vi "chart axis set display units visible.vi"(8 "error in (no error)":errorcluster, 10 "visible":u8, 11 "axis":u32) -> (0 "error out":errorcluster)   [LabVIEW 8.6]
doc: "void chart_axis_set_display_units_visible(lxw_chart_axis axis, uint8_t visible);"
uses:
  pending_lvxlsxwriter/xlsxwriter.dll
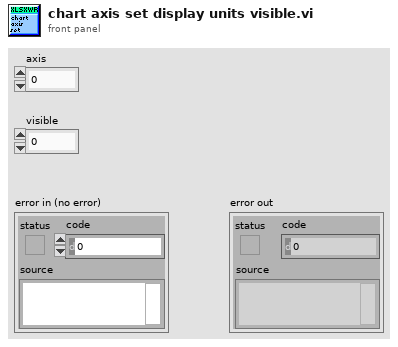
[diagram p1: front panel]
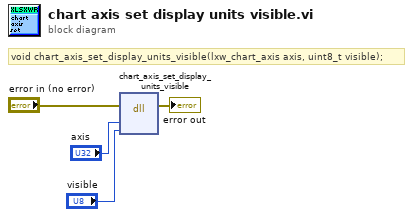
[diagram p0: block diagram]
diagram:
  # "void chart_axis_set_display_units_visible(lxw_chart_axis axis, uint8_t visible);"
  n1 = dll-call lib="C:/Users/WDAGUtilityAccount/Desktop/pending_lvxlsxwriter/xlsxwriter.*" fn="chart_axis_set_display_units_visible"(error in="error in (no error)", "axis"="axis", "visible"="visible") -> (error out=→"error out":errorcluster)  [unwired: 5 in, 1 out]
